vi "Rx Async.vi"(8 "error in (no error)":errorcluster, 11 "Framework in":refnum<class "Framework.lvclass">) -> (0 "error out":errorcluster, 3 "Framework out":refnum<class "Framework.lvclass">)   [LabVIEW 2019, in "DSF Core.lvlib" / "Framework.lvclass"]
uses:
  Framework.lvclass
  Framework.lvclass/Framework.ctl
  Plugin/Plugin.lvclass/Plugin.ctl
  Transfer Group/Transfer Group.lvclass/Transfer Group.ctl
  Timing/Timing.lvclass/Timing.ctl
  Buffers/Buffers.lvclass/Buffers.ctl
  <vilib>/NI/Memory Manager/Classes/Pointer/Pointer.lvclass/Pointer.ctl
  Interface/Interface.lvclass/Interface.ctl
  Transfer Group/Get Iteration and Late Count.vi
  Thread/Dispatcher/Dispatch Transfer Group.vi
  Transfer Group/Get ID.vi
  Transfer Group/Copy Async to Inline.vi
  Transfer Group/Wait For Previous.vi
  Transfer Group/Get Active.vi
  Timing/Get Iteration.vi
  Interface/Dispatcher/Send Dispatcher Command.vi
  Buffers/Copy Async to Inline.vi
  Transfer Group/Retrieve from FIFO.vi
  Transfer Group/Increment Iteration.vi
  Transfer Group/Is Late.vi
  Interface/Dispatcher/Write.vi
  Interface/Dispatcher/Write Dispatcher Command.vi
  <vilib>/NI/Memory Manager/Classes/Pointer/Copy All.vi
  Transfer Group/Read Return FIFO.vi
  Transfer Group/Errors.vi
  Transfer Group/Invalid Iteration Error.vi
  Timing/Increment Iteration.vi
  Transfer Group/Increment Late Count.vi
  Transfer Group/Return Timeout Error.vi
  Interface/Send Command.vi
  Interface/Errors.vi
  Interface/Dispatcher/Command Timeout.vi
  Interface/Dispatcher/Class Name.vi
  <vilib>/NI/Memory Manager/Classes/Pointer/Get Size.vi
  <vilib>/NI/Memory Manager/Classes/Pointer/Copy.vi
  VIs/Constants/Constants.vi
  VIs/Constants/Engine Library Name.vi
  <vilib>/NI/Memory Manager/VIs/New Error Cluster.vi
  <vilib>/NI/Memory Manager/VIs/New Error Cluster (512B).vi
  <vilib>/NI/Memory Manager/VIs/Set Error Status.vi
  <vilib>/NI/Memory Manager/VIs/Set Error Code.vi
  <vilib>/NI/Memory Manager/VIs/Set Error Source.vi
  <vilib>/NI/Memory Manager/VIs/Write String to Source.vi
  <vilib>/NI/Memory Manager/VIs/Write Numeric to Source.vi
  <vilib>/NI/Memory Manager/VIs/Write Numeric Scalar to Source (Base10 U64).vi
  Transfer Group/Transfer Group Error Info.vi
  <vilib>/NI/Memory Manager/VIs/Write Numeric Scalar to Source (Base10 I32).vi
  Interface/Write RT FIFO.vi
  Interface/New Interface Error.vi
  <vilib>/NI/Memory Manager/Classes/Pointer/Copy (No Check).vi
  <vilib>/NI/Memory Manager/Classes/Pointer/Check Bounds (Pointer).vi
  <vilib>/NI/Memory Manager/Classes/Pointer/Check Null Pointer.vi
  VIs/Constants/Base Error Code.vi
  Transfer Group/Transfer Group Error Offset.vi
  Interface/Interface Error Info.vi
  <vilib>/NI/Memory Manager/Classes/Pointer/Get Address.vi
  <vilib>/NI/Memory Manager/Classes/Pointer/Errors.vi
  <vilib>/NI/Memory Manager/Classes/Pointer/Out of Bounds.vi
  <vilib>/NI/Memory Manager/Classes/Pointer/Null Pointer.vi
  <vilib>/NI/Memory Manager/Classes/Pointer/Is Null.vi
  Interface/Interface Error Offset.vi
  <vilib>/NI/Memory Manager/Classes/Pointer/Write Pointer Size to Error.vi
  <vilib>/NI/Memory Manager/Classes/Pointer/Create Error.vi
  <vilib>/NI/Memory Manager/Constants/Constants.vi
  <vilib>/NI/Memory Manager/Constants/Library Name.vi
  <vilib>/NI/Memory Manager/Classes/Pointer/Pointer Error Info.vi
  <vilib>/NI/Memory Manager/Constants/Pointer Class Name.vi
  Buffer/Buffer.lvclass
  C:/Program Files (x86)/National Instruments/LabVIEW 2019/vi.lib/NI/Memory Manager/Classes/Pointer/Pointer.lvclass
  Interface/Dispatcher/Dispatcher Interface.lvclass
  C:/Dev/GitHub/niveristand-data-sharing-framework-custom-device/Core/Classes/Interface/Interface.lvclass
  VIs/VI Name.vi
  Plugin/Plugin.lvclass
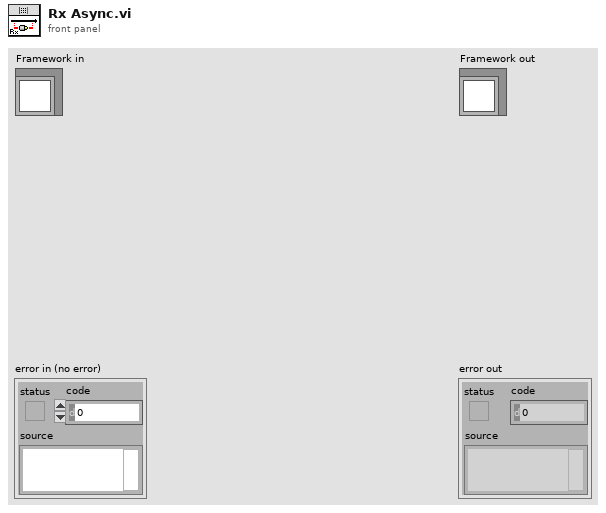
[diagram p1: front panel]
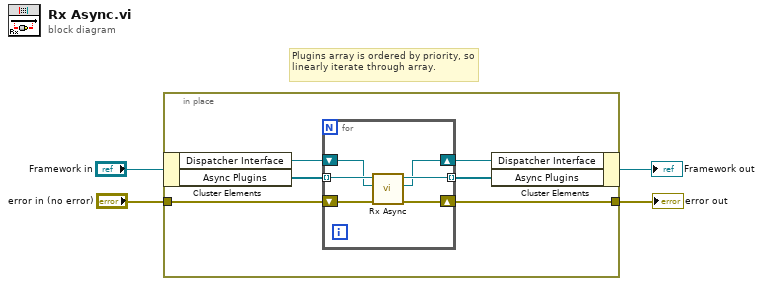
[diagram p0: block diagram]
diagram:
  # "Plugins array is ordered by priority, so linearly iterate through array."
  n1 = in-place {
    in-place-border: "error in (no error)" -> [w10]
    in-place-border: [w9] -> w3
    n2 = in-place-cluster #1("Framework in") -> ("Dispatcher Interface"=w6:refnum<class "Dispatcher Interface.lvclass">, "Async Plugins"=w8:refnum<class "Plugin.lvclass">[])
    n3 = for {
      tunnel: w8 -> [w13] mode=indexing
      tunnel: [w16] -> w7 mode=indexing
      shift-right: [w15] -> w9
      shift-left: w10 -> [w14]
      shift-right: [w11] -> w5
      shift-left: w6 -> [w12]
      n4 = call "Rx Async.vi"("error in (no error)"=w14, "Dispatcher Interface in"=w12, "Plugin in"=w13) -> ("error out"=w15:errorcluster, "Dispatcher Interface out"=w11:refnum<class "Dispatcher Interface.lvclass">, "Plugin out"=w16:refnum<class "Plugin.lvclass">)  [unwired: 6 in]
    }
    n5 = in-place-cluster #1("Dispatcher Interface"=w5, "Async Plugins"=w7) -> (→"Framework out":refnum<class "Framework.lvclass">)
  }
  "error out" <- w3
